vi "ZK_Picturetonumber.vi"(10 "Calibrated Matches 3":T1(array[cluster])=[[{"Position"={"x"=75.99952, "y"=126.03074}, "Angle"=0.0, "Scale"=1.0, "Score"=946.6732, "Bounding Box"=[{"x"=58.99952, "y"=109.03074}, {"x"=91.99952, "y"=109.03074}, {"x"=91.99952, "y"=142.03073}, {"x"=58.99952, "y"=142.03073}, {"x"=58.99952, "y"=109.03074}]}, {"Position"={"x"=279.99457, "y"=228.01927}, "Angle"=0.0, "Scale"=1.0, "Score"=930.5973, "Bounding Box"=[{"x"=262.99457, "y"=211.01927}, {"x"=295.99457, "y"=211.01927}, {"x"=295.99457, "y"=244.01927}, {"x"=262.99457, "y"=244.01927}, {"x"=262.99457, "y"=211.01927}]}, {"Position"={"x"=109.99715, "y"=296.02133}, "Angle"=0.0, "Scale"=1.0, "Score"=922.2777, "Bounding Box"=[{"x"=92.99715, "y"=279.02133}, {"x"=125.99715, "y"=279.02133}, {"x"=125.99715, "y"=312.02133}, {"x"=92.99715, "y"=312.02133}, {"x"=92.99715, "y"=279.02133}]}, {"Position"={"x"=246.00308, "y"=194.01025}, "Angle"=0.0, "Scale"=1.0, "Score"=921.1537, "Bounding Box"=[{"x"=229.00308, "y"=177.01025}, {"x"=262.00308, "y"=177.01025}, {"x"=262.00308, "y"=210.01025}, {"x"=229.00308, "y"=210.01025}, {"x"=229.00308, "y"=177.01025}]}, {"Position"={"x"=245.99716, "y"=296.02094}, "Angle"=0.0, "Scale"=1.0, "Score"=912.61597, "Bounding Box"=[{"x"=228.99716, "y"=279.02094}, {"x"=261.99716, "y"=279.02094}, {"x"=261.99716, "y"=312.02094}, {"x"=228.99716, "y"=312.02094}, {"x"=228.99716, "y"=279.02094}]}, {"Position"={"x"=279.9995, "y"=330.03018}, "Angle"=0.0, "Scale"=1.0, "Score"=912.5403, "Bounding Box"=[{"x"=262.9995, "y"=313.03018}, {"x"=295.9995, "y"=313.03018}, {"x"=295.9995, "y"=346.03018}, {"x"=262.9995, "y"=346.03018}, {"x"=262.9995, "y"=313.03018}]}, {"Position"={"x"=279.99747, "y"=126.0302}, "Angle"=0.0, "Scale"=1.0, "Score"=900.17053, "Bounding Box"=[{"x"=262.99747, "y"=109.0302}, {"x"=295.99747, "y"=109.0302}, {"x"=295.99747, "y"=142.0302}, {"x"=262.99747, "y"=142.0302}, {"x"=262.99747, "y"=109.0302}]}, {"Position"={"x"=109.99351, "y"=364.0303}, "Angle"=0.0, "Scale"=1.0, "Score"=889.1533, "Bounding Box"=[{"x"=92.99351, "y"=347.0303}, {"x"=125.99351, "y"=347.0303}, {"x"=125.99351, "y"=380.0303}, {"x"=92.99351, "y"=380.0303}, {"x"=92.99351, "y"=347.0303}]}, {"Position"={"x"=75.99893, "y"=364.0191}, "Angle"=0.0, "Scale"=1.0, "Score"=880.686, "Bounding Box"=[{"x"=58.99893, "y"=347.0191}, {"x"=91.99893, "y"=347.0191}, {"x"=91.99893, "y"=380.0191}, {"x"=58.99893, "y"=380.0191}, {"x"=58.99893, "y"=347.0191}]}, {"Position"={"x"=0.0, "y"=0.0}, "Angle"=0.0, "Scale"=0.0, "Score"=0.0, "Bounding Box"=[]}, {"Position"={"x"=0.0, "y"=0.0}, "Angle"=0.0, "Scale"=0.0, "Score"=0.0, "Bounding Box"=[]}, {"Position"={"x"=0.0, "y"=0.0}, "Angle"=0.0, "Scale"=0.0, "Score"=0.0, "Bounding Box"=[]}], [{"Position"={"x"=244.93065, "y"=229.00948}, "Angle"=0.0, "Scale"=1.0, "Score"=938.1531, "Bounding Box"=[{"x"=229.93065, "y"=213.00948}, {"x"=258.93066, "y"=213.00948}, {"x"=258.93066, "y"=244.00948}, {"x"=229.93065, "y"=244.00948}, {"x"=229.93065, "y"=213.00948}]}, {"Position"={"x"=177.12814, "y"=229.0155}, "Angle"=0.0, "Scale"=1.0, "Score"=935.3888, "Bounding Box"=[{"x"=162.12814, "y"=213.0155}, {"x"=191.12814, "y"=213.0155}, {"x"=191.12814, "y"=244.0155}, {"x"=162.12814, "y"=244.0155}, {"x"=162.12814, "y"=213.0155}]}, {"Position"={"x"=211.02017, "y"=330.99167}, "Angle"=0.0, "Scale"=1.0, "Score"=932.5707, "Bounding Box"=[{"x"=196.02017, "y"=314.99167}, {"x"=225.02017, "y"=314.99167}, {"x"=225.02017, "y"=345.99167}, {"x"=196.02017, "y"=345.99167}, {"x"=196.02017, "y"=314.99167}]}, {"Position"={"x"=211.03189, "y"=194.98964}, "Angle"=0.0, "Scale"=1.0, "Score"=926.1662, "Bounding Box"=[{"x"=196.03189, "y"=178.98964}, {"x"=225.03189, "y"=178.98964}, {"x"=225.03189, "y"=209.98964}, {"x"=196.03189, "y"=209.98964}, {"x"=196.03189, "y"=178.98964}]}, {"Position"={"x"=177.0608, "y"=297.0077}, "Angle"=0.0, "Scale"=1.0, "Score"=926.0406, "Bounding Box"=[{"x"=162.0608, "y"=281.0077}, {"x"=191.0608, "y"=281.0077}, {"x"=191.0608, "y"=312.0077}, {"x"=162.0608, "y"=312.0077}, {"x"=162.0608, "y"=281.0077}]}, {"Position"={"x"=244.92564, "y"=365.01053}, "Angle"=0.0, "Scale"=1.0, "Score"=925.69135, "Bounding Box"=[{"x"=229.92564, "y"=349.01053}, {"x"=258.92566, "y"=349.01053}, {"x"=258.92566, "y"=380.01053}, {"x"=229.92564, "y"=380.01053}, {"x"=229.92564, "y"=349.01053}]}, {"Position"={"x"=74.99771, "y"=330.99142}, "Angle"=0.0, "Scale"=1.0, "Score"=922.9823, "Bounding Box"=[{"x"=59.99771, "y"=314.99142}, {"x"=88.99771, "y"=314.99142}, {"x"=88.99771, "y"=345.99142}, {"x"=59.99771, "y"=345.99142}, {"x"=59.99771, "y"=314.99142}]}, {"Position"={"x"=108.98091, "y"=161.01422}, "Angle"=0.0, "Scale"=1.0, "Score"=922.14825, "Bounding Box"=[{"x"=93.98091, "y"=145.01422}, {"x"=122.98091, "y"=145.01422}, {"x"=122.98091, "y"=176.01422}, {"x"=93.98091, "y"=176.01422}, {"x"=93.98091, "y"=145.01422}]}, {"Position"={"x"=75.0663, "y"=262.9958}, "Angle"=0.0, "Scale"=1.0, "Score"=921.6964, "Bounding Box"=[{"x"=60.0663, "y"=246.99579}, {"x"=89.0663, "y"=246.99579}, {"x"=89.0663, "y"=277.9958}, {"x"=60.0663, "y"=277.9958}, {"x"=60.0663, "y"=246.99579}]}, {"Position"={"x"=142.96318, "y"=195.01222}, "Angle"=0.0, "Scale"=1.0, "Score"=918.584, "Bounding Box"=[{"x"=127.96318, "y"=179.01222}, {"x"=156.96318, "y"=179.01222}, {"x"=156.96318, "y"=210.01222}, {"x"=127.96318, "y"=210.01222}, {"x"=127.96318, "y"=179.01222}]}, {"Position"={"x"=75.01933, "y"=161.00868}, "Angle"=0.0, "Scale"=1.0, "Score"=910.4724, "Bounding Box"=[{"x"=60.019333, "y"=145.00868}, {"x"=89.01933, "y"=145.00868}, {"x"=89.01933, "y"=176.00868}, {"x"=60.019333, "y"=176.00868}, {"x"=60.019333, "y"=145.00868}]}, {"Position"={"x"=41.14936, "y"=194.99588}, "Angle"=0.0, "Scale"=1.0, "Score"=892.9365, "Bounding Box"=[{"x"=26.14936, "y"=178.99588}, {"x"=55.14936, "y"=178.99588}, {"x"=55.14936, "y"=209.99588}, {"x"=26.14936, "y"=209.99588}, {"x"=26.14936, "y"=178.99588}]}], [{"Position"={"x"=41.057724, "y"=160.01257}, "Angle"=0.0, "Scale"=1.0, "Score"=946.2605, "Bounding Box"=[{"x"=25.057724, "y"=143.01257}, {"x"=56.057724, "y"=143.01257}, {"x"=56.057724, "y"=176.01257}, {"x"=25.057724, "y"=176.01257}, {"x"=25.057724, "y"=143.01257}]}, {"Position"={"x"=211.06906, "y"=296.01663}, "Angle"=0.0, "Scale"=1.0, "Score"=946.0923, "Bounding Box"=[{"x"=195.06906, "y"=279.01663}, {"x"=226.06906, "y"=279.01663}, {"x"=226.06906, "y"=312.01663}, {"x"=195.06906, "y"=312.01663}, {"x"=195.06906, "y"=279.01663}]}, {"Position"={"x"=41.021973, "y"=296.0252}, "Angle"=0.0, "Scale"=1.0, "Score"=944.54456, "Bounding Box"=[{"x"=25.021973, "y"=279.0252}, {"x"=56.021973, "y"=279.0252}, {"x"=56.021973, "y"=312.0252}, {"x"=25.021973, "y"=312.0252}, {"x"=25.021973, "y"=279.0252}]}, {"Position"={"x"=279.0394, "y"=364.10086}, "Angle"=0.0, "Scale"=1.0, "Score"=934.75385, "Bounding Box"=[{"x"=263.0394, "y"=347.10086}, {"x"=294.0394, "y"=347.10086}, {"x"=294.0394, "y"=380.10086}, {"x"=263.0394, "y"=380.10086}, {"x"=263.0394, "y"=347.10086}]}, {"Position"={"x"=108.919014, "y"=330.02905}, "Angle"=0.0, "Scale"=1.0, "Score"=931.9961, "Bounding Box"=[{"x"=92.919014, "y"=313.02905}, {"x"=123.919014, "y"=313.02905}, {"x"=123.919014, "y"=346.02905}, {"x"=92.919014, "y"=346.02905}, {"x"=92.919014, "y"=313.02905}]}, {"Position"={"x"=244.95236, "y"=160.01564}, "Angle"=0.0, "Scale"=1.0, "Score"=916.7709, "Bounding Box"=[{"x"=228.95236, "y"=143.01564}, {"x"=259.95236, "y"=143.01564}, {"x"=259.95236, "y"=176.01564}, {"x"=228.95236, "y"=176.01564}, {"x"=228.95236, "y"=143.01564}]}, {"Position"={"x"=143.11177, "y"=330.03476}, "Angle"=0.0, "Scale"=1.0, "Score"=915.4203, "Bounding Box"=[{"x"=127.11177, "y"=313.03476}, {"x"=158.11177, "y"=313.03476}, {"x"=158.11177, "y"=346.03476}, {"x"=127.11177, "y"=346.03476}, {"x"=127.11177, "y"=313.03476}]}, {"Position"={"x"=109.091484, "y"=194.12073}, "Angle"=0.0, "Scale"=1.0, "Score"=913.47217, "Bounding Box"=[{"x"=93.091484, "y"=177.12073}, {"x"=124.091484, "y"=177.12073}, {"x"=124.091484, "y"=210.12073}, {"x"=93.091484, "y"=210.12073}, {"x"=93.091484, "y"=177.12073}]}, {"Position"={"x"=245.13066, "y"=126.00052}, "Angle"=0.0, "Scale"=1.0, "Score"=910.05774, "Bounding Box"=[{"x"=229.13066, "y"=109.00052}, {"x"=260.13068, "y"=109.00052}, {"x"=260.13068, "y"=142.00052}, {"x"=229.13066, "y"=142.00052}, {"x"=229.13066, "y"=109.00052}]}, {"Position"={"x"=41.04156, "y"=364.03253}, "Angle"=0.0, "Scale"=1.0, "Score"=902.44653, "Bounding Box"=[{"x"=25.041561, "y"=347.03253}, {"x"=56.04156, "y"=347.03253}, {"x"=56.04156, "y"=380.03253}, {"x"=25.041561, "y"=380.03253}, {"x"=25.041561, "y"=347.03253}]}, {"Position"={"x"=0.0, "y"=0.0}, "Angle"=0.0, "Scale"=0.0, "Score"=0.0, "Bounding Box"=[]}, {"Position"={"x"=0.0, "y"=0.0}, "Angle"=0.0, "Scale"=0.0, "Score"=0.0, "Bounding Box"=[]}], [{"Position"={"x"=246.03236, "y"=328.80533}, "Angle"=0.0, "Scale"=1.0, "Score"=952.347, "Bounding Box"=[{"x"=231.03236, "y"=312.80533}, {"x"=261.03235, "y"=312.80533}, {"x"=261.03235, "y"=343.80533}, {"x"=231.03236, "y"=343.80533}, {"x"=231.03236, "y"=312.80533}]}, {"Position"={"x"=212.07097, "y"=158.96404}, "Angle"=0.0, "Scale"=1.0, "Score"=952.17175, "Bounding Box"=[{"x"=197.07097, "y"=142.96404}, {"x"=227.07097, "y"=142.96404}, {"x"=227.07097, "y"=173.96404}, {"x"=197.07097, "y"=173.96404}, {"x"=197.07097, "y"=142.96404}]}, {"Position"={"x"=177.95842, "y"=125.27156}, "Angle"=0.0, "Scale"=1.0, "Score"=950.7424, "Bounding Box"=[{"x"=162.95842, "y"=109.27156}, {"x"=192.95842, "y"=109.27156}, {"x"=192.95842, "y"=140.27156}, {"x"=162.95842, "y"=140.27156}, {"x"=162.95842, "y"=109.27156}]}, {"Position"={"x"=144.06927, "y"=125.20636}, "Angle"=0.0, "Scale"=1.0, "Score"=929.157, "Bounding Box"=[{"x"=129.06927, "y"=109.20636}, {"x"=159.06927, "y"=109.20636}, {"x"=159.06927, "y"=140.20636}, {"x"=129.06927, "y"=140.20636}, {"x"=129.06927, "y"=109.20636}]}, {"Position"={"x"=0.0, "y"=0.0}, "Angle"=0.0, "Scale"=0.0, "Score"=0.0, "Bounding Box"=[]}, {"Position"={"x"=0.0, "y"=0.0}, "Angle"=0.0, "Scale"=0.0, "Score"=0.0, "Bounding Box"=[]}, {"Position"={"x"=0.0, "y"=0.0}, "Angle"=0.0, "Scale"=0.0, "Score"=0.0, "Bounding Box"=[]}, {"Position"={"x"=0.0, "y"=0.0}, "Angle"=0.0, "Scale"=0.0, "Score"=0.0, "Bounding Box"=[]}, {"Position"={"x"=0.0, "y"=0.0}, "Angle"=0.0, "Scale"=0.0, "Score"=0.0, "Bounding Box"=[]}, {"Position"={"x"=0.0, "y"=0.0}, "Angle"=0.0, "Scale"=0.0, "Score"=0.0, "Bounding Box"=[]}, {"Position"={"x"=0.0, "y"=0.0}, "Angle"=0.0, "Scale"=0.0, "Score"=0.0, "Bounding Box"=[]}, {"Position"={"x"=0.0, "y"=0.0}, "Angle"=0.0, "Scale"=0.0, "Score"=0.0, "Bounding Box"=[]}], [{"Position"={"x"=142.99628, "y"=260.98865}, "Angle"=0.0, "Scale"=1.0, "Score"=926.0769, "Bounding Box"=[{"x"=126.99628, "y"=244.98865}, {"x"=158.99628, "y"=244.98865}, {"x"=158.99628, "y"=276.98865}, {"x"=126.99628, "y"=276.98865}, {"x"=126.99628, "y"=244.98865}]}, {"Position"={"x"=278.96713, "y"=295.00446}, "Angle"=0.0, "Scale"=1.0, "Score"=914.9557, "Bounding Box"=[{"x"=262.96713, "y"=279.00446}, {"x"=294.96713, "y"=279.00446}, {"x"=294.96713, "y"=311.00446}, {"x"=262.96713, "y"=311.00446}, {"x"=262.96713, "y"=279.00446}]}, {"Position"={"x"=176.98276, "y"=193.00453}, "Angle"=0.0, "Scale"=1.0, "Score"=912.5583, "Bounding Box"=[{"x"=160.98276, "y"=177.00453}, {"x"=192.98276, "y"=177.00453}, {"x"=192.98276, "y"=209.00453}, {"x"=160.98276, "y"=209.00453}, {"x"=160.98276, "y"=177.00453}]}, {"Position"={"x"=108.97621, "y"=260.9978}, "Angle"=0.0, "Scale"=1.0, "Score"=909.02466, "Bounding Box"=[{"x"=92.97621, "y"=244.9978}, {"x"=124.97621, "y"=244.9978}, {"x"=124.97621, "y"=276.9978}, {"x"=92.97621, "y"=276.9978}, {"x"=92.97621, "y"=244.9978}]}, {"Position"={"x"=142.97182, "y"=159.00162}, "Angle"=0.0, "Scale"=1.0, "Score"=897.2611, "Bounding Box"=[{"x"=126.97182, "y"=143.00162}, {"x"=158.97182, "y"=143.00162}, {"x"=158.97182, "y"=175.00162}, {"x"=126.97182, "y"=175.00162}, {"x"=126.97182, "y"=143.00162}]}, {"Position"={"x"=76.0, "y"=227.0}, "Angle"=0.0, "Scale"=1.0, "Score"=888.2339, "Bounding Box"=[{"x"=60.0, "y"=211.0}, {"x"=92.0, "y"=211.0}, {"x"=92.0, "y"=243.0}, {"x"=60.0, "y"=243.0}, {"x"=60.0, "y"=211.0}]}, {"Position"={"x"=210.98383, "y"=363.03317}, "Angle"=0.0, "Scale"=1.0, "Score"=881.3889, "Bounding Box"=[{"x"=194.98383, "y"=347.03317}, {"x"=226.98383, "y"=347.03317}, {"x"=226.98383, "y"=379.03317}, {"x"=194.98383, "y"=379.03317}, {"x"=194.98383, "y"=347.03317}]}, {"Position"={"x"=211.01735, "y"=125.01166}, "Angle"=0.0, "Scale"=1.0, "Score"=868.12415, "Bounding Box"=[{"x"=195.01735, "y"=109.01166}, {"x"=227.01735, "y"=109.01166}, {"x"=227.01735, "y"=141.01166}, {"x"=195.01735, "y"=141.01166}, {"x"=195.01735, "y"=109.01166}]}, {"Position"={"x"=143.01091, "y"=363.00833}, "Angle"=0.0, "Scale"=1.0, "Score"=850.3575, "Bounding Box"=[{"x"=127.01091, "y"=347.00833}, {"x"=159.01091, "y"=347.00833}, {"x"=159.01091, "y"=379.00833}, {"x"=127.01091, "y"=379.00833}, {"x"=127.01091, "y"=347.00833}]}, {"Position"={"x"=29.181082, "y"=223.97372}, "Angle"=0.0, "Scale"=1.0, "Score"=802.54517, "Bounding Box"=[{"x"=13.181082, "y"=207.97372}, {"x"=45.181084, "y"=207.97372}, {"x"=45.181084, "y"=239.97372}, {"x"=13.181082, "y"=239.97372}, {"x"=13.181082, "y"=207.97372}]}, {"Position"={"x"=0.0, "y"=0.0}, "Angle"=0.0, "Scale"=0.0, "Score"=0.0, "Bounding Box"=[]}, {"Position"={"x"=0.0, "y"=0.0}, "Angle"=0.0, "Scale"=0.0, "Score"=0.0, "Bounding Box"=[]}], [{"Position"={"x"=144.09454, "y"=295.99463}, "Angle"=0.0, "Scale"=1.0, "Score"=935.2221, "Bounding Box"=[{"x"=128.09454, "y"=278.99463}, {"x"=159.09454, "y"=278.99463}, {"x"=159.09454, "y"=312.99463}, {"x"=128.09454, "y"=312.99463}, {"x"=128.09454, "y"=278.99463}]}, {"Position"={"x"=41.628357, "y"=330.0011}, "Angle"=0.0, "Scale"=1.0, "Score"=929.2328, "Bounding Box"=[{"x"=25.628357, "y"=313.0011}, {"x"=56.628357, "y"=313.0011}, {"x"=56.628357, "y"=347.0011}, {"x"=25.628357, "y"=347.0011}, {"x"=25.628357, "y"=313.0011}]}, {"Position"={"x"=177.78041, "y"=261.98907}, "Angle"=0.0, "Scale"=1.0, "Score"=926.96277, "Bounding Box"=[{"x"=161.78041, "y"=244.98907}, {"x"=192.78041, "y"=244.98907}, {"x"=192.78041, "y"=278.98907}, {"x"=161.78041, "y"=278.98907}, {"x"=161.78041, "y"=244.98907}]}, {"Position"={"x"=211.9815, "y"=262.03052}, "Angle"=0.0, "Scale"=1.0, "Score"=921.9062, "Bounding Box"=[{"x"=195.9815, "y"=245.03052}, {"x"=226.9815, "y"=245.03052}, {"x"=226.9815, "y"=279.03052}, {"x"=195.9815, "y"=279.03052}, {"x"=195.9815, "y"=245.03052}]}, {"Position"={"x"=41.770508, "y"=125.98808}, "Angle"=0.0, "Scale"=1.0, "Score"=918.2764, "Bounding Box"=[{"x"=25.770508, "y"=108.98808}, {"x"=56.770508, "y"=108.98808}, {"x"=56.770508, "y"=142.98808}, {"x"=25.770508, "y"=142.98808}, {"x"=25.770508, "y"=108.98808}]}, {"Position"={"x"=143.91397, "y"=227.98573}, "Angle"=0.0, "Scale"=1.0, "Score"=913.74005, "Bounding Box"=[{"x"=127.91397, "y"=210.98573}, {"x"=158.91397, "y"=210.98573}, {"x"=158.91397, "y"=244.98573}, {"x"=127.91397, "y"=244.98573}, {"x"=127.91397, "y"=210.98573}]}, {"Position"={"x"=177.63574, "y"=329.998}, "Angle"=0.0, "Scale"=1.0, "Score"=911.9823, "Bounding Box"=[{"x"=161.63574, "y"=312.998}, {"x"=192.63574, "y"=312.998}, {"x"=192.63574, "y"=346.998}, {"x"=161.63574, "y"=346.998}, {"x"=161.63574, "y"=312.998}]}, {"Position"={"x"=109.9738, "y"=125.992165}, "Angle"=0.0, "Scale"=1.0, "Score"=905.7056, "Bounding Box"=[{"x"=93.9738, "y"=108.992165}, {"x"=124.9738, "y"=108.992165}, {"x"=124.9738, "y"=142.99216}, {"x"=93.9738, "y"=142.99216}, {"x"=93.9738, "y"=108.992165}]}, {"Position"={"x"=178.02208, "y"=160.01111}, "Angle"=0.0, "Scale"=1.0, "Score"=891.8085, "Bounding Box"=[{"x"=162.02208, "y"=143.01111}, {"x"=193.02208, "y"=143.01111}, {"x"=193.02208, "y"=177.01111}, {"x"=162.02208, "y"=177.01111}, {"x"=162.02208, "y"=143.01111}]}, {"Position"={"x"=280.09894, "y"=159.99469}, "Angle"=0.0, "Scale"=1.0, "Score"=885.4157, "Bounding Box"=[{"x"=264.09894, "y"=142.99469}, {"x"=295.09894, "y"=142.99469}, {"x"=295.09894, "y"=176.99469}, {"x"=264.09894, "y"=176.99469}, {"x"=264.09894, "y"=142.99469}]}, {"Position"={"x"=177.99521, "y"=364.00534}, "Angle"=0.0, "Scale"=1.0, "Score"=880.8915, "Bounding Box"=[{"x"=161.99521, "y"=347.00534}, {"x"=192.99521, "y"=347.00534}, {"x"=192.99521, "y"=381.00534}, {"x"=161.99521, "y"=381.00534}, {"x"=161.99521, "y"=347.00534}]}, {"Position"={"x"=0.0, "y"=0.0}, "Angle"=0.0, "Scale"=0.0, "Score"=0.0, "Bounding Box"=[]}], [{"Position"={"x"=40.981247, "y"=262.00372}, "Angle"=0.0, "Scale"=1.0, "Score"=901.4845, "Bounding Box"=[{"x"=23.981247, "y"=245.00372}, {"x"=57.981247, "y"=245.00372}, {"x"=57.981247, "y"=279.00372}, {"x"=23.981247, "y"=279.00372}, {"x"=23.981247, "y"=245.00372}]}, {"Position"={"x"=244.99156, "y"=262.00342}, "Angle"=0.0, "Scale"=1.0, "Score"=896.3923, "Bounding Box"=[{"x"=227.99156, "y"=245.00342}, {"x"=261.99158, "y"=245.00342}, {"x"=261.99158, "y"=279.00342}, {"x"=227.99156, "y"=279.00342}, {"x"=227.99156, "y"=245.00342}]}, {"Position"={"x"=108.952705, "y"=228.00728}, "Angle"=0.0, "Scale"=1.0, "Score"=893.5738, "Bounding Box"=[{"x"=91.952705, "y"=211.00728}, {"x"=125.952705, "y"=211.00728}, {"x"=125.952705, "y"=245.00728}, {"x"=91.952705, "y"=245.00728}, {"x"=91.952705, "y"=211.00728}]}, {"Position"={"x"=278.9555, "y"=262.0003}, "Angle"=0.0, "Scale"=1.0, "Score"=890.87756, "Bounding Box"=[{"x"=261.9555, "y"=245.0003}, {"x"=295.9555, "y"=245.0003}, {"x"=295.9555, "y"=279.0003}, {"x"=261.9555, "y"=279.0003}, {"x"=261.9555, "y"=245.0003}]}, {"Position"={"x"=210.99438, "y"=228.00267}, "Angle"=0.0, "Scale"=1.0, "Score"=882.012, "Bounding Box"=[{"x"=193.99438, "y"=211.00267}, {"x"=227.99438, "y"=211.00267}, {"x"=227.99438, "y"=245.00267}, {"x"=193.99438, "y"=245.00267}, {"x"=193.99438, "y"=211.00267}]}, {"Position"={"x"=75.00315, "y"=296.0069}, "Angle"=0.0, "Scale"=1.0, "Score"=877.1368, "Bounding Box"=[{"x"=58.00315, "y"=279.0069}, {"x"=92.00315, "y"=279.0069}, {"x"=92.00315, "y"=313.0069}, {"x"=58.00315, "y"=313.0069}, {"x"=58.00315, "y"=279.0069}]}, {"Position"={"x"=278.9641, "y"=193.99812}, "Angle"=0.0, "Scale"=1.0, "Score"=875.59357, "Bounding Box"=[{"x"=261.9641, "y"=176.99812}, {"x"=295.9641, "y"=176.99812}, {"x"=295.9641, "y"=210.99812}, {"x"=261.9641, "y"=210.99812}, {"x"=261.9641, "y"=176.99812}]}, {"Position"={"x"=0.0, "y"=0.0}, "Angle"=0.0, "Scale"=0.0, "Score"=0.0, "Bounding Box"=[]}, {"Position"={"x"=0.0, "y"=0.0}, "Angle"=0.0, "Scale"=0.0, "Score"=0.0, "Bounding Box"=[]}, {"Position"={"x"=0.0, "y"=0.0}, "Angle"=0.0, "Scale"=0.0, "Score"=0.0, "Bounding Box"=[]}, {"Position"={"x"=0.0, "y"=0.0}, "Angle"=0.0, "Scale"=0.0, "Score"=0.0, "Bounding Box"=[]}, {"Position"={"x"=0.0, "y"=0.0}, "Angle"=0.0, "Scale"=0.0, "Score"=0.0, "Bounding Box"=[]}]]) -> (2 "Array":dbl[][](array[numeric])=[[0.0, 1.0, 0.0, 0.0, 0.0, 0.0, 0.0, 1.0], [0.0, 0.0, 0.0, 0.0, 0.0, 0.0, 0.0, 0.0], [0.0, 0.0, 0.0, 0.0, 0.0, 0.0, 1.0, 0.0], [0.0, 0.0, 0.0, 0.0, 0.0, 0.0, 0.0, 1.0], [0.0, 0.0, 0.0, 0.0, 0.0, 0.0, 0.0, 0.0], [0.0, 0.0, 1.0, 0.0, 0.0, 0.0, 1.0, 0.0], [0.0, 0.0, 0.0, 0.0, 0.0, 0.0, 0.0, 1.0], [0.0, 1.0, 1.0, 0.0, 0.0, 0.0, 0.0, 0.0]])   [LabVIEW 2018]
panel:
  out "Numeric":i32=11
  out "Cluster":T2
  # "Animal"
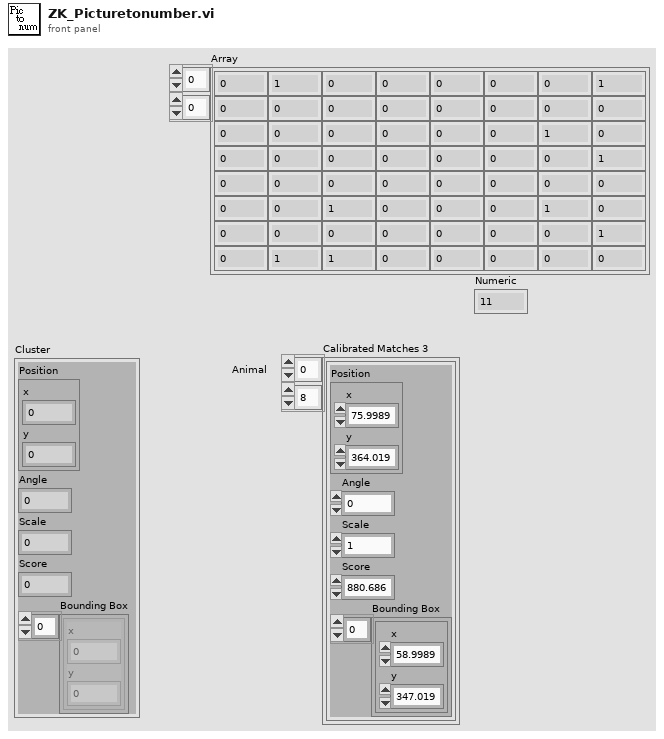
[diagram p1: front panel]
types:
  T1 = cluster{"Position":cluster{"x":sgl, "y":sgl}, "Angle":sgl, "Scale":sgl, "Score":sgl, "Bounding Box":cluster{"x":sgl, "y":sgl}[]}[][]
  T2 = cluster{"Position":cluster{"x":sgl, "y":sgl}, "Angle":sgl, "Scale":sgl, "Score":sgl, "Bounding Box":cluster{"x":sgl, "y":sgl}[]}
  T3 = cluster{"LU_X":i32, "LU_Y":i32, "RD_X":i32, "RD_Y":i32}
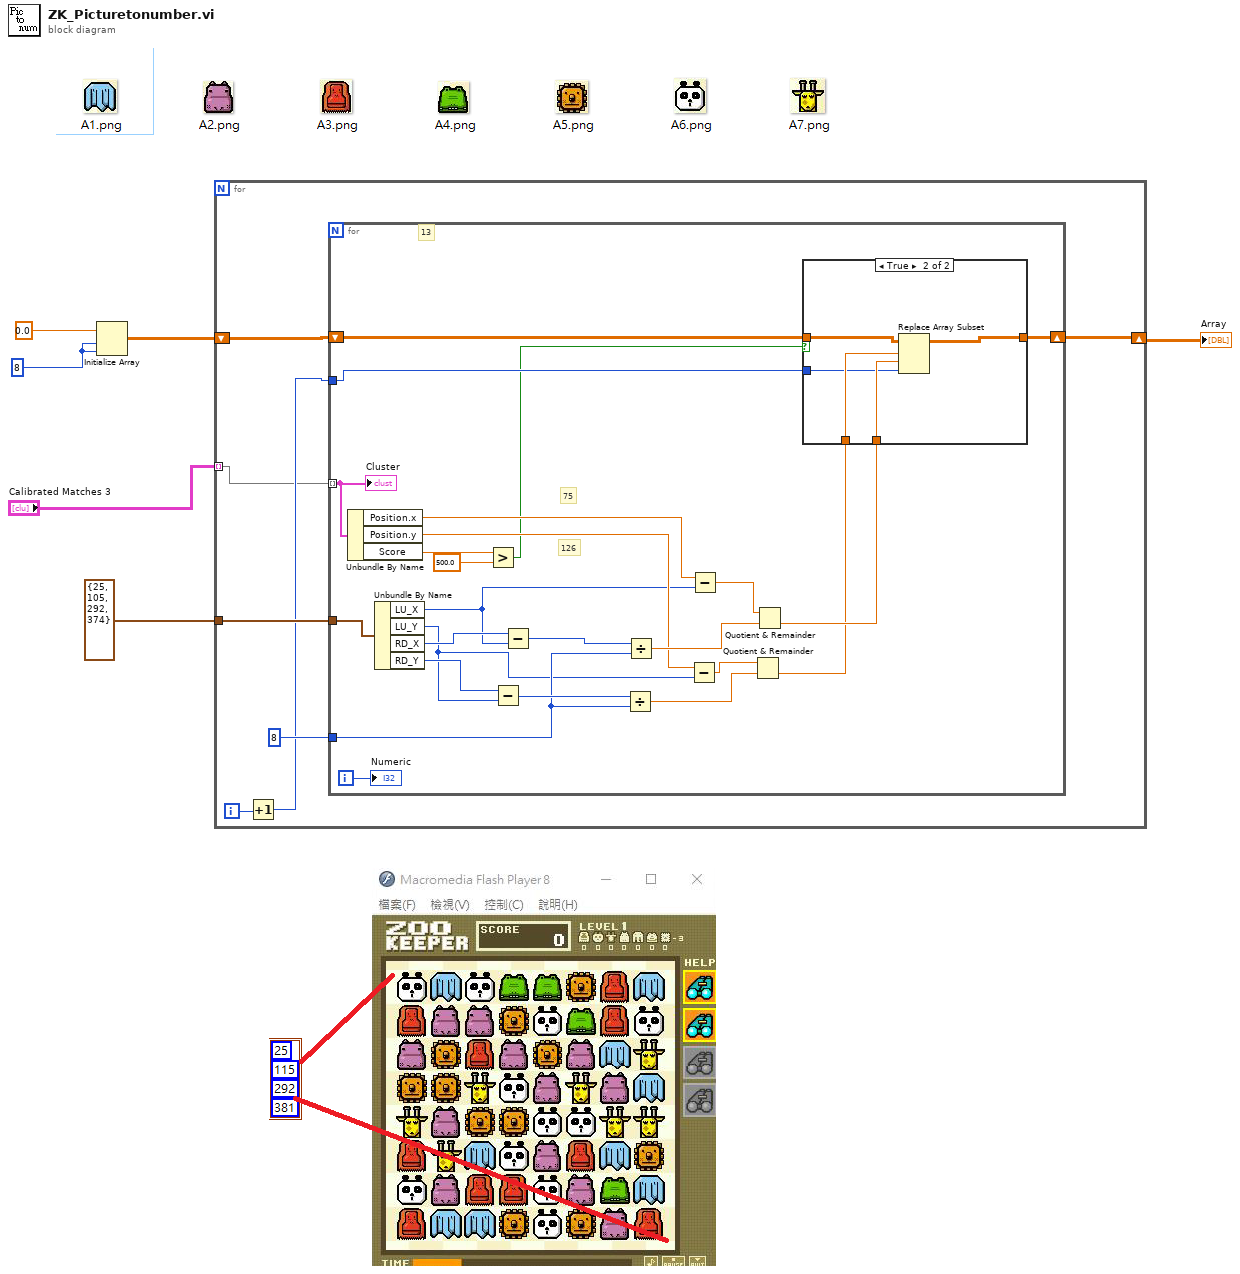
[diagram p0: block diagram]
diagram:
  w5 = 8 ("dimension size")
  n1 = Initialize Array "Initialize Array"(0.0 ("element"), w5, w5) -> (w3:dbl[][])
  n2 = for {
    tunnel: T3 {"LU_X"=25, "LU_Y"=105, "RD_X"=292, "RD_Y"=374} ("Cluster 2") -> [w13]
    tunnel: "Calibrated Matches 3" -> [w7] mode=indexing
    shift-right: [w10] -> w2
    shift-left: w3 -> [w11]
    i -> [w9]
    n3 = Increment(x=w9) -> (x+1=w8:i32)
    n4 = for {
      tunnel: w7 -> [w36] mode=indexing
      tunnel: w13 -> [w35]
      tunnel: 8 -> [w32]
      tunnel: w8 -> [w29]
      shift-right: [w31] -> w10
      shift-left: w11 -> [w30]
      i -> [w37]
      # "126"
      # "75"
      # "13"
      n5 = Unbundle By Name(w36) -> ("Position.x"=w28:sgl, "Position.y"=w25:sgl, "Score"=w22:sgl)
      n6 = Unbundle By Name(w35) -> ("LU_X"=w17:i32, "LU_Y"=w16:i32, "RD_X"=w19:i32, "RD_Y"=w18:i32)
      n7 = Greater?(x=w22, y=sgl 500.0) -> (0:w20:bool)
      n8 = Subtract(x=w18, y=w16) -> (x-y=w33:i32)
      n9 = Subtract(x=w19, y=w17) -> (x-y=w34:i32)
      n10 = Divide(x=w33, y=w32) -> (x/y=w24:dbl)
      n11 = Divide(x=w34, y=w32) -> (x/y=w27:dbl)
      n12 = Subtract(x=w25, y=w16) -> (x-y=w23:sgl)
      n13 = Subtract(x=w28, y=w17) -> (x-y=w26:sgl)
      n14 = Quotient & Remainder(x=w23, y=w24) -> (floor(x/y)=w14:dbl)  [unwired: 1 out]
      n15 = Quotient & Remainder(x=w26, y=w27) -> (floor(x/y)=w15:dbl)  [unwired: 1 out]
      n16 = case shown="True" w20 {
        tunnel: [w38 w43] -> w31
        tunnel: w30 -> [w38 w42]
        tunnel: w14 -> [_ w41]
        tunnel: w15 -> [_ w40]
        tunnel: w29 -> [_ w39]
        frame False {
        }
        frame True {
          n17 = Replace Array Subset "Replace Array Subset"(array=w42, new element=w39, index (row)=w41, index (col)=w40) -> (w43:dbl[][])
        }
      }
      "Cluster" <- w36
      "Numeric" <- w37
    }
  }
  "Array" <- w2
